vi "Directional Transform (SubVI).vi"(10 "Transform Amount (mm)":dbl=-100.0 format="%#_13g", 11 "Pose":cluster{"X":dbl, "Y":dbl, "R":dbl}) -> (3 "Pose":cluster{"X":dbl, "Y":dbl, "R":dbl})   [LabVIEW 2017]
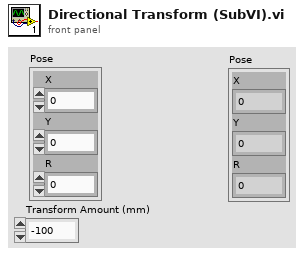
[diagram p1: front panel]
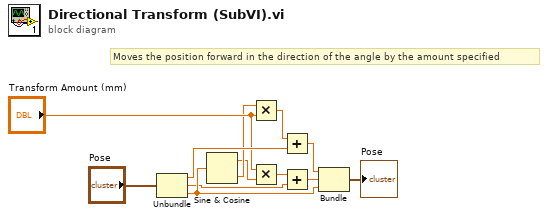
[diagram p0: block diagram]
diagram:
  # "Moves the position forward in the direction of the angle by the amount specified"
  n1 = Unbundle("Pose") -> ("X"=w7:dbl, "Y"=w8:dbl, "R"=w12:dbl)
  n2 = Sine & Cosine(0:w12) -> (1:w2:dbl, 2:w3:dbl)
  n3 = Multiply(x=w3, y="Transform Amount (mm)") -> (x*y=w6:dbl)
  n4 = Multiply(x="Transform Amount (mm)", y=w2) -> (x*y=w9:dbl)
  n5 = Add(x=w6, y=w7) -> (x+y=w10:dbl)
  n6 = Add(x=w9, y=w8) -> (x+y=w11:dbl)
  n7 = Bundle(w10, w11, "R"=w12) -> (→"Pose":cluster{dbl, dbl, "R":dbl})  [unwired: 1 in]
